vi "Initialize.vi"(7 "Channel Name":string="Setpoint.ch%d.SP", 8 "error in":errorcluster, 9 "Number of Channels":u32=1, 10 "Instance Name":string="PluginName", 11 "Flow Gradient in":refnum<class "Flow Gradient.lvclass">) -> (0 "error out":errorcluster, 2 "Channel":T1[](array[typedef]), 3 "Flow Gradient out":refnum<class "Flow Gradient.lvclass">)   [LabVIEW 2023, in "Flow Gradient.lvclass"]
uses:
  Flow Gradient.lvclass
  Parents/Gradient/Gradient.lvclass
  Utilities/Channel.ctl
  Utilities/Utilities.lvlib
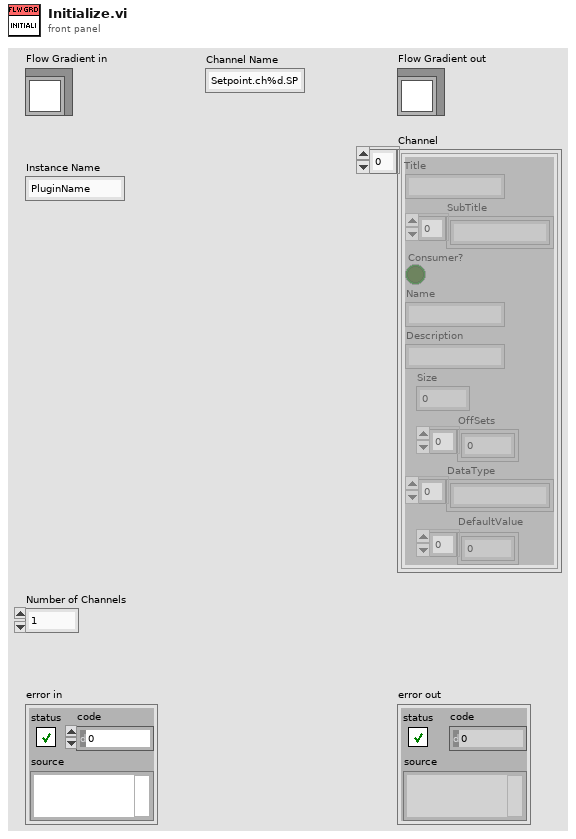
[diagram p1: front panel]
types:
  T1 = typedef "Utilities.lvlib/Channel.ctl" = cluster{"Title":string, "SubTitle":string[], "Consumer?":bool, "Name":string, "Description":string, "Size":i32, "OffSets":i32[], "DataType":string[], "DefaultValue":dbl[]}
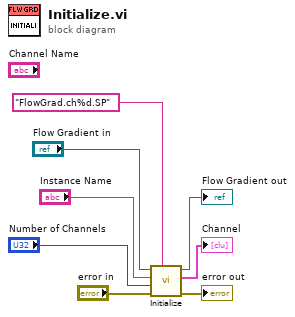
[diagram p0: block diagram]
diagram:
  n1 = call-parent "Initialize.vi"("Channel Name"="FlowGrad.ch%d.SP", "error in"="error in", "Number of Channels"="Number of Channels", "Instance Name"="Instance Name", "Gradient in"="Flow Gradient in") -> ("error out"=→"error out":errorcluster, "Channel"=→"Channel":T1[], "Gradient out"=→"Flow Gradient out":refnum<class "Flow Gradient.lvclass">)  [unwired: 4 in]
